vi "Entrain2.vi"() -> ()   [LabVIEW 2012]
uses:
  <vilib>/Platform/TimedLoop/XDataNode/XDataNode.xnode
  <vilib>/Platform/TimedLoop/XDataNode/nitl_modes.ctl
  <vilib>/Platform/TimedLoop/XDataNode/XDNodeRunTimeDep.lvlib
  <vilib>/Platform/TimedLoop/XDataNode/wakeup.ctl
  <vilib>/Platform/TimedLoop/XDataNode/timing_clust.ctl
  Treatment.ctl
  Data.ctl
  Treatment type.ctl
  <vilib>/Analysis/3filter.llb/Filter Passband Type.ctl
  <vilib>/Analysis/NI_AALBase.lvlib
panel:
  out "Actual Start [i]":i64
  out "Cur noise":dbl caption="Noise amplitude (deg)"
  out "Cur amp":dbl caption="Stimulus amplitude (deg)"
  out "R":dbl[](array[numeric])
  out "mean phase":dbl[](array[numeric])
  in  "reset phase":bool
  out "Cur freq":dbl caption="Stimulus frequency (Hz)"
  out "PSD":cluster{"f0":dbl, "df":dbl, "magnitude":dbl[]}[](graph)
  in  "Threshold":dbl=0.1
  out "Sweep":cluster{cluster{dbl, dbl}[]}[](graph)
  out "Raw data":waveform(dbl)[](graph)
  in  "Stop":bool
  out "Data file":path
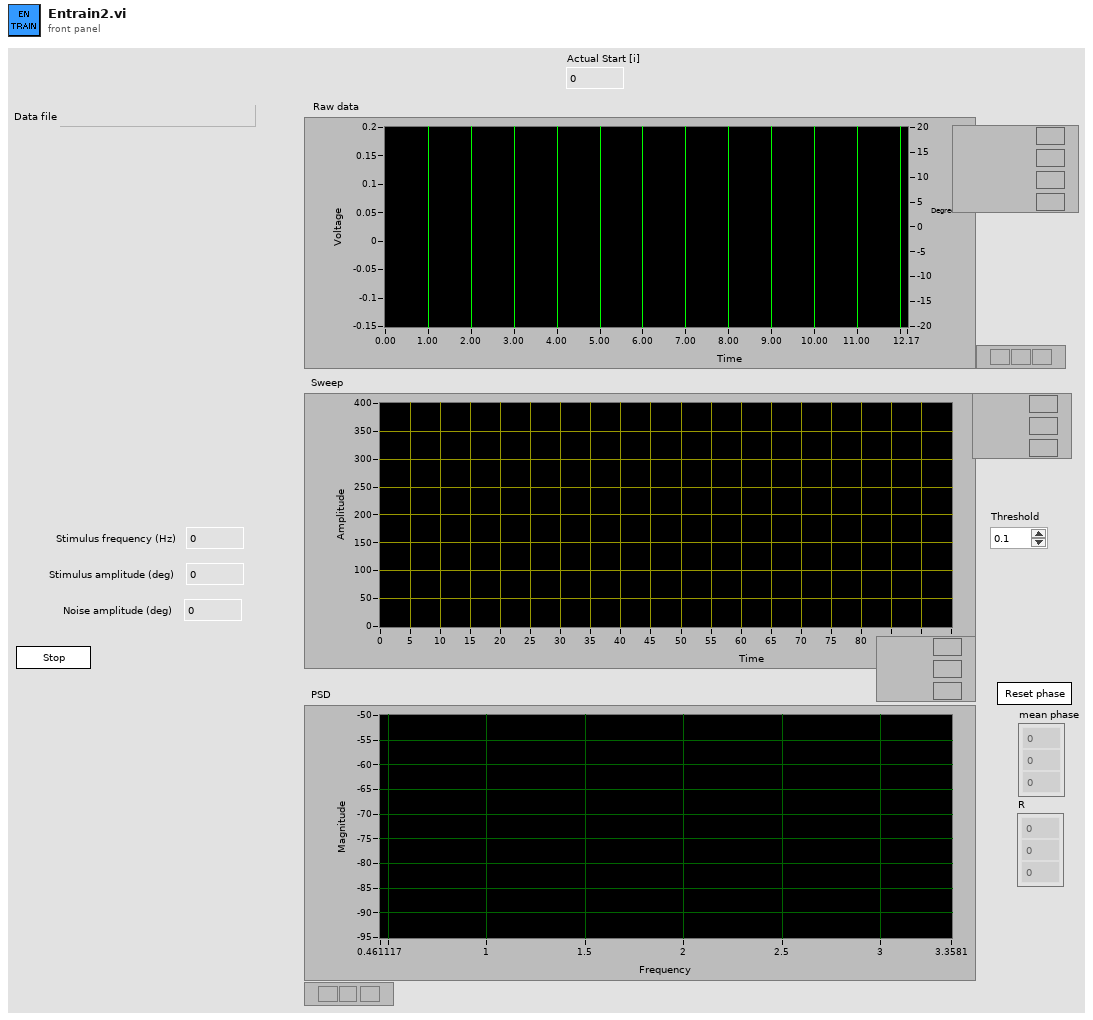
[diagram p1: front panel]
types:
  T1 = typedef "Treatment.ctl" = cluster{"sample":dbl, "startphase":dbl, "type":T2, "frequency":dbl, "amplitude":dbl, "noise":dbl, "duration":dbl, "kfreq":dbl, "noisehifreq":dbl, "frequency2":dbl, "amplitude2":dbl, "startphase2":dbl, "noise filter type":T3, "noiselofreq":dbl, "amp change":dbl, "noise change":dbl}
  T2 = typedef "Treatment type.ctl" = enum16{"Zero", "Sine", "Frequency sweep", "Two frequency", "Amplitude sweep"}
  T3 = typedef "NI_AALBase.lvlib/Filter Passband Type.ctl" = enum32{"Lowpass", "Highpass", "Bandpass", "Bandstop"}
  T4 = typedef "Sampling info.ctl" = cluster{"Channels":T5[], "Sampling freq":i32, "Output freq":i32, "Update freq":i32, "Steps per rev":i32, "Counts per rev":i32, "Amplifier":string, "Motor driver":string, "Step bit":u8, "Max speed":dbl, "Max accel":dbl, "Pos gain":dbl, "Vel gain":dbl, "counter":tag}
  T5 = typedef "Channel.ctl" = cluster{"Name":string, "Chan":tag, "Gain":u16, "Lo cutoff":dbl, "Hi cutoff":dbl, "Notch":bool}
  T6 = typedef "Data.ctl" = cluster{"Voltage data":dbl[][], "Encoder data":dbl[], "Motor output":dbl[], "Current treatment":T1, "Motor speed":dbl[], "Clipped motor":dbl[], "new treatment":bool}
  T7 = typedef "File refs.ctl" = cluster{"file":T8, "voltage data":i32, "motor data":i32, "command data":i32, "encoder data":i32}
  T8 = typedef "hid_t.ctl" = i32
  T9 = typedef "Run info.ctl" = cluster{"voltage task":refnum<k21>, "dummy output task":refnum<k21>, "digital output task":refnum<k21>, "encoder task":refnum<k21>, "n input samples":i32, "n output samples":i32, "max speed":dbl, "max accel":dbl, "last pos":dbl, "last vel":dbl, "pos gain":dbl, "vel gain":dbl, "input dt":dbl, "output freq":dbl}
  T10 = typedef "XDNodeRunTimeDep.lvlib/timing_clust.ctl" = cluster{"Expected End [f-1]":u64, "Actual End [f-1]":u64, "Finished Late? [f-1]":bool, "Expected End [i-1]":u64, "Actual End [i-1]":u64, "Finished Late? [i-1]":bool, "Expected Start [i]":u64, "Actual Start [i]":u64, "Expected Start [f]":u64, "Actual Start [f]":u64, "Source Name":string, "Structure Name":string, "Period":i64, "Deadline":i64, "Offset":i64, "Start":i64, "Priority":i32, "Timeout":i32, "Mode":T11, "Wakeup Reason":T12, "Error":errorcluster, "Source Type":string, "Secondary Source Type":string, "Global End Time":u64, "Global Start Time":u64, "Frame Duration":u64, "Iteration Duration":u64, "Assigned CPU":i32, "I/O Scan Engine Mode":u32}
  T11 = typedef "XDNodeRunTimeDep.lvlib/nitl_modes.ctl" = enum32{"No Change", "Process missed periods, maintain original phase", "Discard missed periods, maintain original phase", "Process missed periods, ignore original phase", "Discard missed periods, ignore original phase"}
  T12 = typedef "XDNodeRunTimeDep.lvlib/wakeup.ctl" = enum32{"Normal", "Aborted", "Asynchronous wakeup", "Timing source error", "Timed loop error", "Timeout"}
  T13 = typedef "Motor Cmd.ctl" = cluster{"stepper cmd":u32[], "servo cmd":cluster{"duty cycle":dbl, "frequency":dbl}[]}
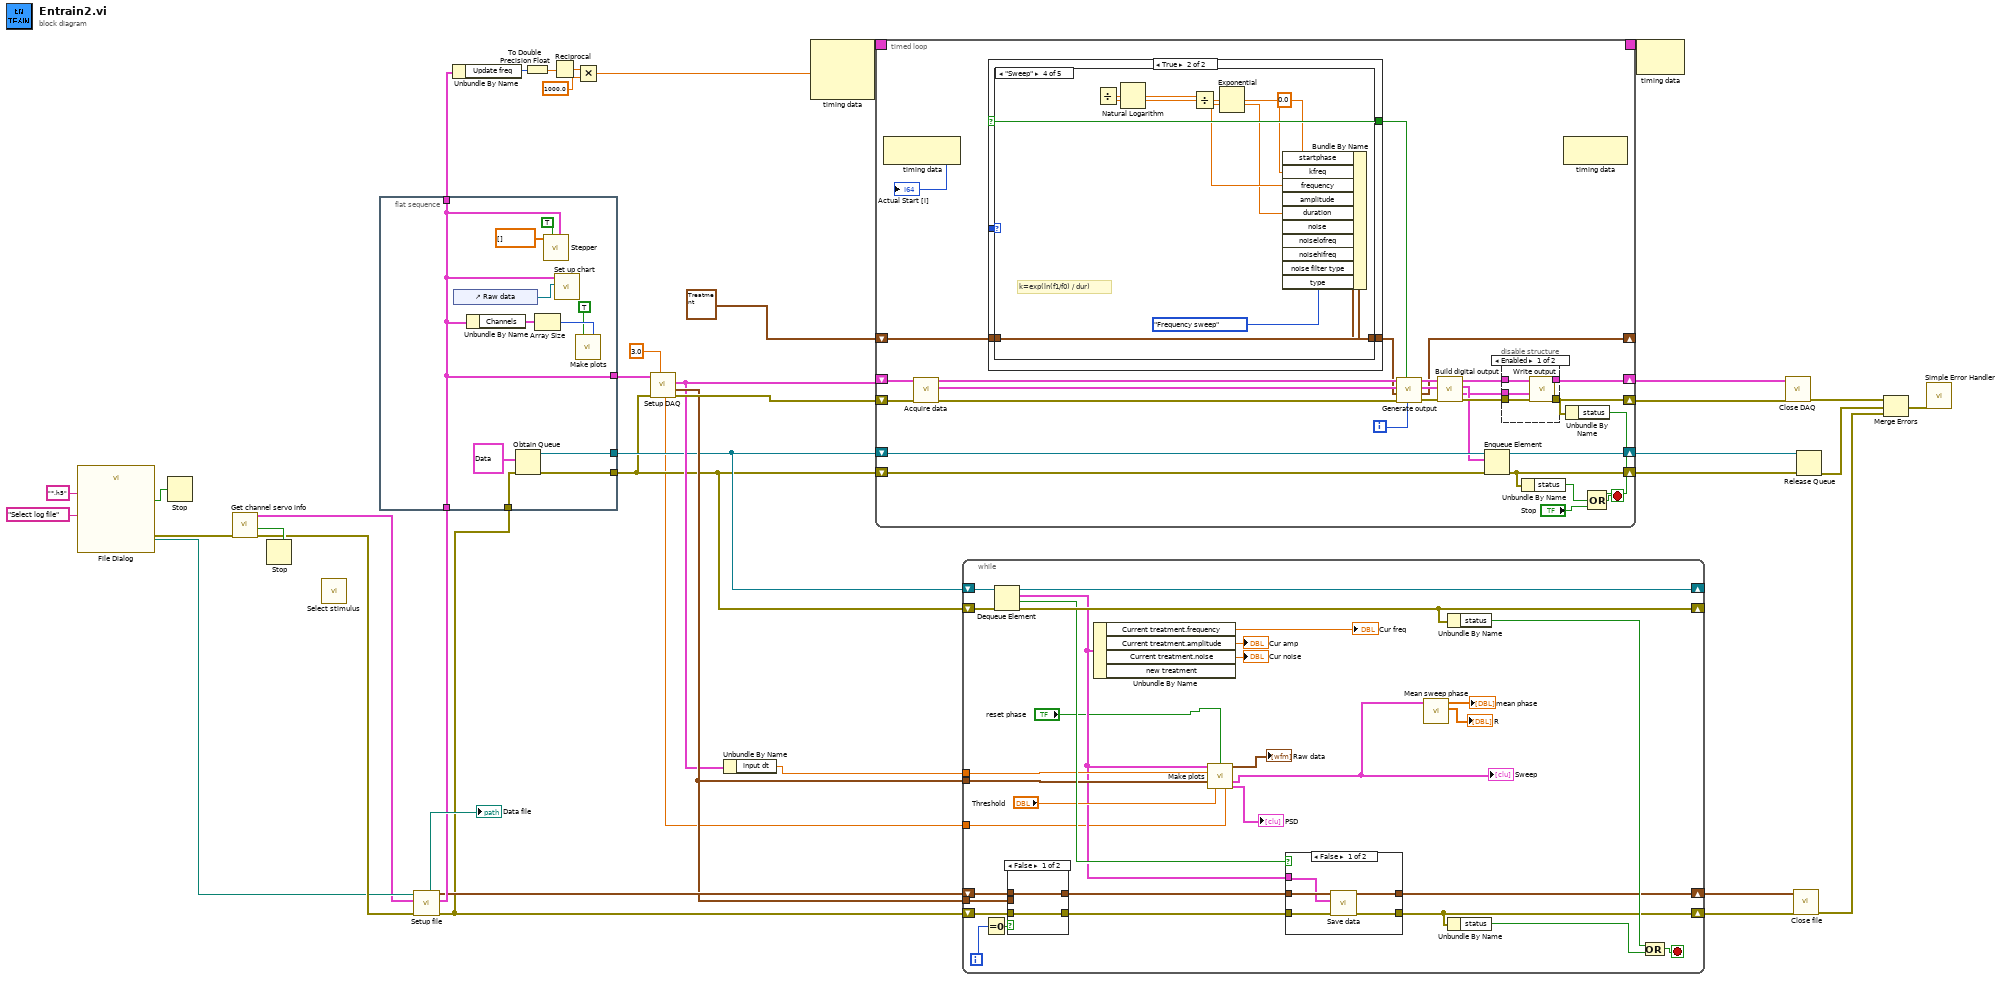
[diagram p0: block diagram]
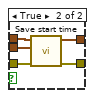
[diagram p2: hidden frame]
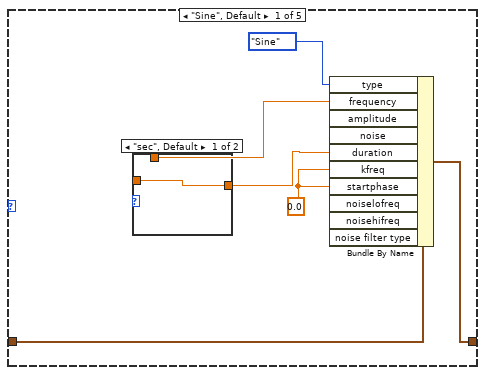
[diagram p6: hidden frame]
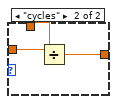
[diagram p7: hidden frame]
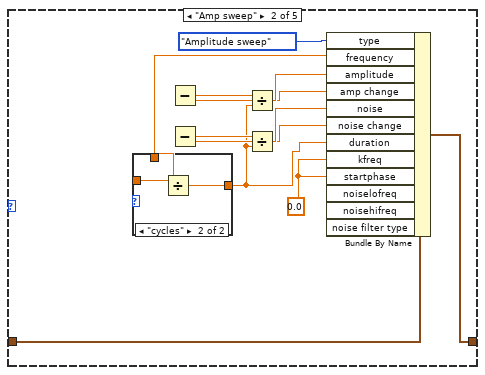
[diagram p8: hidden frame]
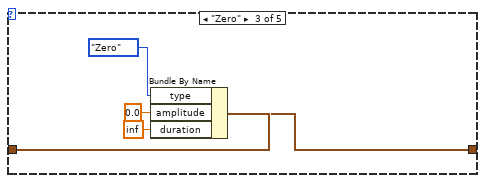
[diagram p10: hidden frame]
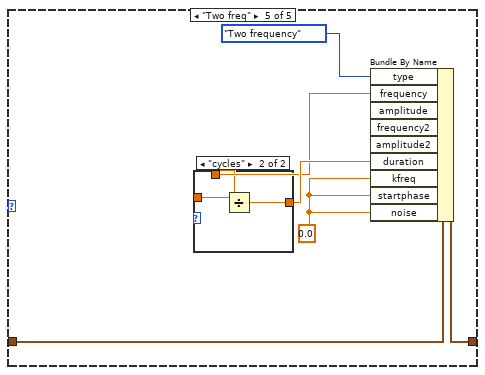
[diagram p11: hidden frame]
diagram:
  n1 = call "File Dialog"("prompt"="Select log file", "pattern (all files)"="*.h5") -> ("selected path"=w35:path, "cancelled"=w38:bool, "error out"=w34:errorcluster)  [unwired: 10 in, 1 out]
  n2 = Stop(stop? (T)=w38) -> ()
  n3 = call "Get channel servo info.vi"("error in"=w34) -> ("error out"=w36:errorcluster, "Cancelled"=w37:bool, "Sampling info"=w33:T4)  [unwired: 8 in]
  n4 = Stop(stop? (T)=w37) -> ()
  n5 = call "Select stimulus.vi"() -> ()  [unwired: 8 in, 3 out]
  n6 = flat-sequence {
    tunnel: [w49] -> w4
    tunnel: w12 -> [w41]
    tunnel: [w43] -> w3
    tunnel: w10 -> [w42]
    tunnel: [w41] -> w8
    tunnel: [w41] -> w7
    frame #0 {
      n7 = control-ref of="Raw data"() -> (w47:refnum<vi>)
      n8 = Unbundle By Name(w41) -> ("Channels"=w46:T5[])
      n9 = Obtain Queue(element data type=T6 {"Voltage data"=[], "Encoder data"=[], "Motor output"=[], "Current treatment"={"sample"=0.0, "startphase"=0.0, "type"=enum."Zero", "frequency"=0.0, "amplitude"=0.0, "noise"=0.0, "duration"=0.0, "kfreq"=0.0, "noisehifreq"=0.0, "frequency2"=0.0, "amplitude2"=0.0, "startphase2"=0.0, "noise filter type"=enum."Lowpass", "noiselofreq"=0.0, "amp change"=0.0, "noise change"=0.0}, "Motor speed"=[], "Clipped motor"=[], "new treatment"=FALSE} ("Data"), error in (no error)=w42) -> (queue out=w49:refnum<queue>, error out=w43:errorcluster)  [unwired: 3 in, 1 out]
      n10 = Array Size(array=w46) -> (size(s)=w45:i32)
      n11 = call "Stepper.vi"("Sampling info"=w41, "initialize"=TRUE, "position"=dbl[] []) -> ()  [unwired: 7 in, 2 out]
      n12 = call "Set up chart.vi"("chart reference"=w47, "Sampling data"=w41) -> ()  [unwired: 10 in]
      n13 = call "Make plots.vi"("init"=TRUE, "nchan"=w45) -> ()  [unwired: 11 in, 3 out]
    }
  }
  n14 = call "Setup file.vi"("error in (no error)"=w36, "Sampling data"=w33, "selected path"=w35) -> ("error out"=w10:errorcluster, "Sampling data out"=w12:T4, "file refs"=w11:T7, "path out"=→"Data file":path)  [unwired: 5 in]
  n15 = Unbundle By Name(w8) -> ("Update freq"=w30:i32)
  n16 = To Double Precision Float(number=w30) -> (double precision float=w29:dbl)
  n17 = Reciprocal(x=w29) -> (1/x=w28:dbl)
  n18 = Multiply(x=w28, y=1000.0) -> (x*y=w15:dbl)
  n19 = call "Setup DAQ.vi"("buffer size multiple"=3.0, "error in (no error)"=w3, "Sampling info in"=w7) -> ("error out"=w14:errorcluster, "start time"=w9:timestamp, "Run info"=w5:T9, "output delay"=w2:dbl)  [unwired: 4 in, 1 out]
  n20 = Unbundle By Name(w5) -> ("input dt"=w13:dbl)
  n21 = node-c288(w15) -> (w32:T10)  [unwired: 2 in]
  n22 = timed-loop {
    timing: w32 -> [_]
    timing-out: [_] -> w31
    shift-right: [w61] -> _
    shift-left: T1 {"sample"=0.0, "startphase"=0.0, "type"=enum."Zero", "frequency"=0.0, "amplitude"=0.0, "noise"=0.0, "duration"=inf, "kfreq"=0.0, "noisehifreq"=20.0, "frequency2"=0.0, "amplitude2"=0.0, "startphase2"=0.0, "noise filter type"=enum."Lowpass", "noiselofreq"=0.0, "amp change"=0.0, "noise change"=0.0} ("Current treatment") -> [w57]
    shift-right: [w74] -> w18
    shift-left: w14 -> [w81]
    shift-right: [w73] -> w24
    shift-left: w3 -> [w76]
    shift-right: [w75] -> w17
    shift-left: w5 -> [w82]
    shift-right: [w68] -> w25
    shift-left: w4 -> [w77]
    i -> [w62]
    stop <- w70 stop-if-true
    n23 = node-c288() -> (→"Actual Start [i]":i64)  [unwired: 1 in]
    n24 = call "Acquire data.vi"("error in"=w81, "Run info"=w82) -> ("error out"=w78:errorcluster, "Data out"=w79:T6, "Run info out"=w80:T9)  [unwired: 7 in]
    n25 = case shown="True" w58 {
      selector: [w90 w92] -> w58
      tunnel: [_ w95] -> w59
      tunnel: w57 -> [w91 w94]
      tunnel: [w91 w93] -> w56
      tunnel: [w90 w92] -> w55
      frame False {
      }
      frame True {
        n26 = case shown="\"Sweep\"" w95 {
          tunnel: w94 -> [w102 w126 w133 w144 w159]
          tunnel: [w101 w125 w132 w143 w154] -> w93
          frame "Sine", Default {
            w99 = 0.0 ("kfreq")
            n27 = case shown="\"sec\", Default" {
              selector: _ -> [_ _]
              tunnel: _ -> [w107 w110]
              tunnel: w104 -> [_ w109]
              tunnel: [w107 w108] -> w103
              frame "sec", Default {
              }
              frame "cycles" {
                n28 = Divide(x=w110, y=w109) -> (x/y=w108:dbl)
              }
            }
            n29 = Bundle By Name(cluster=w102, "type"=Treatment_type."Sine", "duration"=w103, "kfreq"=w99, "startphase"=w99) -> (w101:T1, "frequency"=w104:dbl, "amplitude"=w106:dbl, "noise"=w105:dbl, "noiselofreq"=w98:dbl, "noisehifreq"=w97:dbl, "noise filter type"=w96:T3)
          }
          frame "Amp sweep" {
            w123 = 0.0 ("kfreq")
            n30 = case shown="\"cycles\"" {
              selector: _ -> [_ _]
              tunnel: _ -> [w128 w131]
              tunnel: w127 -> [_ w130]
              tunnel: [w128 w129] -> w112
              frame "sec", Default {
              }
              frame "cycles" {
                n31 = Divide(x=w131, y=w130) -> (x/y=w129:dbl)
              }
            }
            n32 = Subtract(y=w118) -> (x=w119:dbl, x-y=w117:dbl)
            n33 = Divide(x=w117, y=w112) -> (x/y=w116:dbl)
            n34 = Subtract(y=w114) -> (x=w115:dbl, x-y=w113:dbl)
            n35 = Divide(x=w113, y=w112) -> (x/y=w111:dbl)
            n36 = Bundle By Name(cluster=w126, "type"=Treatment_type."Amplitude sweep", "amp change"=w116, "noise change"=w111, "duration"=w112, "kfreq"=w123, "startphase"=w123) -> (w125:T1, "frequency"=w127:dbl, "amplitude"=w118:dbl, "noise"=w114:dbl, "noiselofreq"=w122:dbl, "noisehifreq"=w121:dbl, "noise filter type"=w120:T3)
          }
          frame "Zero" {
            n37 = Bundle By Name(cluster=w133, "type"=Treatment_type."Zero", "amplitude"=0.0, "duration"=inf) -> (w132:T1)
          }
          frame "Sweep" {
            # "k=exp(ln(f1/f0) / dur)"
            n38 = Divide() -> (x=w148:dbl, y=w147:dbl, x/y=w152:dbl)
            n39 = Natural Logarithm(1:w152) -> (0:w151:dbl)
            n40 = Divide(x=w151, y=w142) -> (x/y=w150:dbl)
            n41 = Exponential(1:w150) -> (0:w149:dbl)
            n42 = Bundle By Name(cluster=w144, "startphase"=0.0, "kfreq"=w149, "frequency"=w147, "type"=Treatment_type."Frequency sweep") -> (w143:T1, "amplitude"=w146:dbl, "duration"=w142:dbl, "noise"=w140:dbl, "noiselofreq"=w139:dbl, "noisehifreq"=w138:dbl, "noise filter type"=w137:T3)
          }
          frame "Two freq" {
            w153 = 0.0 ("kfreq")
            n43 = case shown="\"cycles\"" w156 {
              tunnel: [w164 w167] -> w155
              tunnel: [_ w166] -> w161
              tunnel: [w164 w165] -> w163
              frame "sec", Default {
              }
              frame "cycles" {
                n44 = Divide(x=w167, y=w166) -> (x/y=w165:dbl)
              }
            }
            n45 = Bundle By Name(cluster=w159, "type"=Treatment_type."Two frequency", "frequency"=w161, "duration"=w163, "kfreq"=w153, "startphase"=w153, "noise"=w153) -> (w154:T1, "amplitude"=w160:dbl, "frequency2"=w158:dbl, "amplitude2"=w157:dbl)
          }
        }
      }
    }
    n46 = call "Generate output.vi"("index"=w62, "new treatment"=w55, "error in"=w78, "Current treatment"=w56, "Data in"=w79, "Run info"=w80) -> ("error out"=w63:errorcluster, "Current treatment out"=w61:T1, "Data out"=w67:T6, "Run info out"=w66:T9)  [unwired: 2 in]
    n47 = call "Build digital output.vi"("error in"=w63, "Data in"=w67, "Run info"=w66) -> ("error out"=w64:errorcluster, "Motor cmd"=w53:T13, "Data out"=w60:T6, "Run info out"=w65:T9, "enable"=w54:bool)  [unwired: 4 in]
    n48 = Enqueue Element(queue=w77, element=w60, error in (no error)=w76) -> (queue out=w68:refnum<queue>, error out=w73:errorcluster)  [unwired: 1 in, 1 out]
    n49 = disable-structure shown="Enabled" {
      disable-tunnel: [w87 w89] -> w75
      disable-tunnel: [w86 w88] -> w74
      disable-tunnel: w65 -> [w85 w89]
      disable-tunnel: w64 -> [w84 w88]
      disable-tunnel: w53 -> [w83 _]
      frame Enabled {
        n50 = call "Write output.vi"("error in"=w84, "data"=w83, "Run info"=w85) -> ("error out"=w86:errorcluster, "Run info out"=w87:T9)  [unwired: 7 in]
      }
      frame Disabled {
      }
    }
    n51 = Unbundle By Name(w73) -> ("status"=w71:bool)
    n52 = node-c288() -> ()  [unwired: 1 in, 1 out]
    n53 = Unbundle By Name(w74) -> ("status"=w72:bool)
    n54 = Compound Arithmetic op=OR(w72, w71, "Stop") -> (w70:bool)
  }
  n55 = while {
    shift-right: [w201] -> _
    shift-left: w3 -> [w195]
    shift-right: [w194] -> w23
    shift-left: w11 -> [w184]
    shift-right: [w193] -> w22
    shift-left: w10 -> [w182]
    shift-right: [w197] -> _
    shift-left: w4 -> [w196]
    tunnel: w9 -> [w191]
    tunnel: w13 -> [w189]
    tunnel: w9 -> [w187]
    tunnel: w2 -> [w177]
    i -> [w186]
    stop <- w200 stop-if-true
    n56 = Equal To 0?(x=w186) -> (x = 0?=w185:bool)
    n57 = Dequeue Element(queue=w196, error in (no error)=w195) -> (queue out=w197:refnum<queue>, element=w179:T6, timed out?=w192:bool, error out=w201:errorcluster)  [unwired: 1 in]
    n58 = case shown="False" w185 {
      tunnel: w187 -> [_ w208]
      tunnel: w184 -> [w203 w207]
      tunnel: [w203 w206] -> w183
      tunnel: w182 -> [w202 w205]
      tunnel: [w202 w204] -> w181
      frame False {
      }
      frame True {
        n59 = call "Save start time.vi"("error in (no error)"=w205, "Start time"=w208, "file refs"=w207) -> ("error out"=w204:errorcluster, "file refs out"=w206:T7)  [unwired: 7 in]
      }
    }
    n60 = Unbundle By Name(w179) -> ("Current treatment.frequency"=→"Cur freq":dbl, "Current treatment.amplitude"=→"Cur amp":dbl, "Current treatment.noise"=→"Cur noise":dbl)  [unwired: 1 out]
    n61 = call "Make plots.vi"("Data in"=w179, "reset phase"="reset phase", "dt"=w189, "start time"=w191, "threshold"="Threshold", "output delay"=w177) -> ("plot data"=→"Raw data":waveform(dbl)[], "Sweep data"=w176:cluster{cluster{dbl, dbl}[]}[], "PSD"=→"PSD":cluster{"f0":dbl, "df":dbl, "magnitude":dbl[]}[])  [unwired: 7 in]
    "Sweep" <- w176
    n62 = case shown="False" w192 {
      tunnel: w183 -> [w213 w215]
      tunnel: w181 -> [w212 w214]
      tunnel: w179 -> [w209 _]
      tunnel: [w211 w215] -> w194
      tunnel: [w210 w214] -> w193
      frame False {
        n63 = call "Save data.vi"("error in (no error)"=w212, "Data"=w209, "file refs"=w213) -> ("error out"=w210:errorcluster, "file refs out"=w211:T7)  [unwired: 7 in]
      }
      frame True {
      }
    }
    n64 = call "Mean sweep phase.vi"("Sweep data"=w176) -> ("R"=→"R":dbl[], "Mean phase"=→"mean phase":dbl[])  [unwired: 9 in]
    n65 = Unbundle By Name(w201) -> ("status"=w199:bool)
    n66 = Unbundle By Name(w193) -> ("status"=w198:bool)
    n67 = Compound Arithmetic op=OR(w199, w198) -> (w200:bool)
  }
  n68 = node-c288(w31) -> ()  [unwired: 1 out]
  n69 = call "Close DAQ.vi"("error in"=w18, "Run info"=w17) -> ("error out"=w16:errorcluster)  [unwired: 9 in]
  n70 = call "Close file.vi"("error in (no error)"=w22, "file refs"=w23) -> ("error out"=w20:errorcluster)  [unwired: 9 in]
  n71 = Release Queue(queue=w25, error in (no error)=w24) -> (error out=w21:errorcluster)  [unwired: 1 in, 2 out]
  n72 = Merge Errors(w16, w21, w20) -> (w19:errorcluster)
  n73 = call <vilib>:"Simple Error Handler.vi"("error in (no error)"=w19) -> ()  [unwired: 4 in, 5 out]
